vi "Accelerometer_Standalone.vi"() -> ()   [LabVIEW 2025]
uses:
  <vilib>/Instr/_visa.llb/VISA Configure Serial Port (Instr).vi
panel:
  in  "RESET":bool
  in  "Serial Port":refnum<visa-resource-name>="COM8"
  out "ACC7":cluster{"OUTX":dbl, "OUTY":dbl, "OUTZ":dbl}
  out "ACC6":cluster{"OUTX":dbl, "OUTY":dbl, "OUTZ":dbl}
  out "ACC5":cluster{"OUTX":dbl, "OUTY":dbl, "OUTZ":dbl}
  out "ACC4":cluster{"OUTX":dbl, "OUTY":dbl, "OUTZ":dbl}
  out "ACC3":cluster{"OUTX":dbl, "OUTY":dbl, "OUTZ":dbl}
  out "ACC2":cluster{"OUTX":dbl, "OUTY":dbl, "OUTZ":dbl}
  out "ACC1":cluster{"OUTX":dbl, "OUTY":dbl, "OUTZ":dbl}
  out "ACC0":cluster{"OUTX":dbl, "OUTY":dbl, "OUTZ":dbl}
  out "ACC7":cluster{"OUTX":dbl, "OUTY":dbl, "OUTZ":dbl}(graph)
  out "ACC6":cluster{"OUTX":dbl, "OUTY":dbl, "OUTZ":dbl}(graph)
  out "ACC5":cluster{"OUTX":dbl, "OUTY":dbl, "OUTZ":dbl}(graph)
  out "ACC4":cluster{"OUTX":dbl, "OUTY":dbl, "OUTZ":dbl}(graph)
  out "ACC3":cluster{"OUTX":dbl, "OUTY":dbl, "OUTZ":dbl}(graph)
  out "ACC2":cluster{"OUTX":dbl, "OUTY":dbl, "OUTZ":dbl}(graph)
  out "ACC1":cluster{"OUTX":dbl, "OUTY":dbl, "OUTZ":dbl}(graph)
  out "ACC0":cluster{"OUTX":dbl, "OUTY":dbl, "OUTZ":dbl}(graph)
  in  "Z7":dbl
  in  "Y7":dbl
  in  "X7":dbl
  in  "Z6":dbl
  in  "Y6":dbl
  in  "X6":dbl
  in  "Z5":dbl
  in  "Y5":dbl
  in  "X5":dbl
  in  "Z4":dbl=0.9
  in  "Y4":dbl=-0.18
  in  "X4":dbl=-0.05
  in  "Z3":dbl=0.9
  in  "Y3":dbl
  in  "X3":dbl
  in  "Z2":dbl=0.7
  in  "Y2":dbl=0.55
  in  "X2":dbl=0.05
  in  "Z1":dbl
  in  "Y1":dbl
  in  "X1":dbl
  in  "Z0":dbl
  in  "Y0":dbl
  in  "X0":dbl
  out "error out":errorcluster
  in  "Continous Run":bool=TRUE
  # "ACC 1 Correction Factor"
  # "ACC 0 Correction Factor"
  # "ACC 3 Correction Factor"
  # "ACC 2 Correction Factor"
  # "ACC 5 Correction Factor"
  # "ACC 4 Correction Factor"
  # "ACC 7 Correction Factor"
  # "ACC 6 Correction Factor"
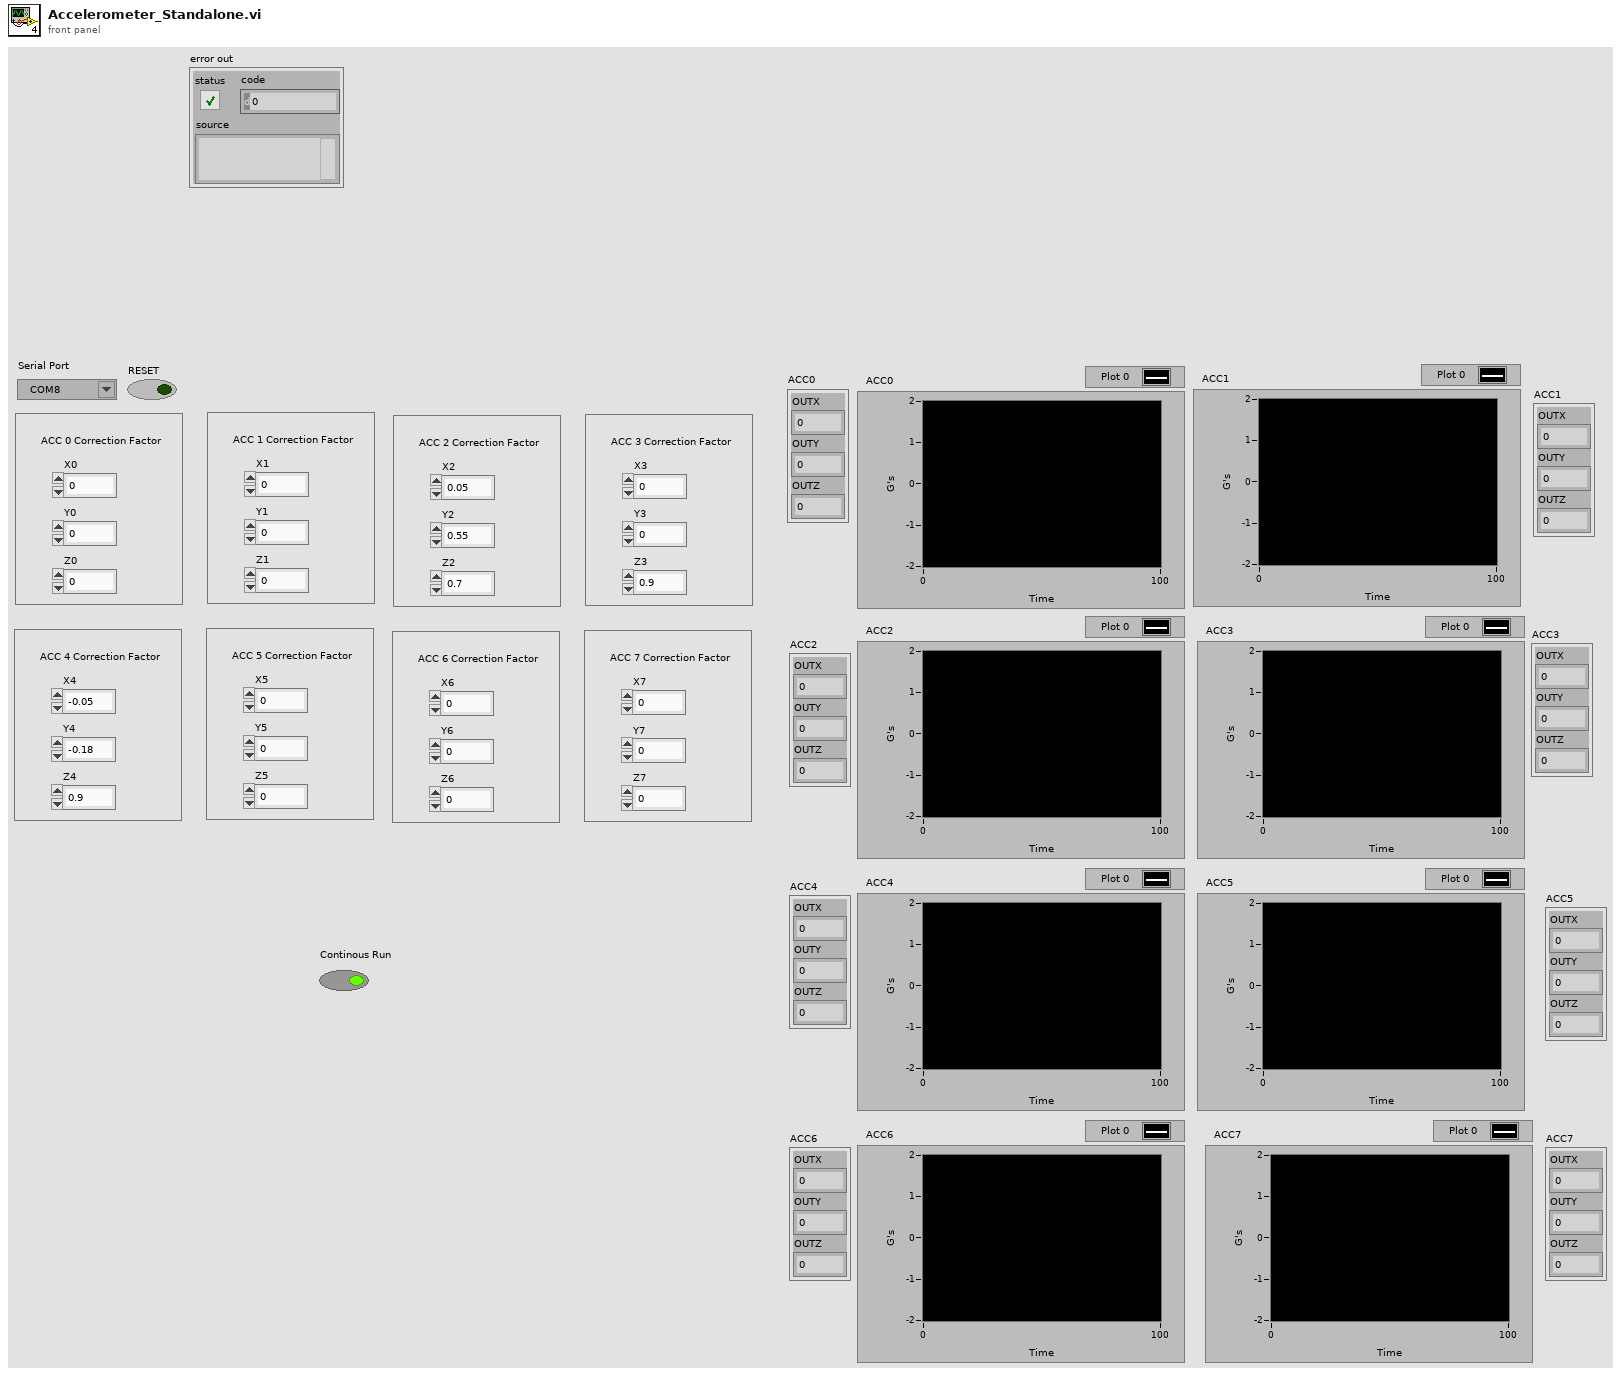
[diagram p1: front panel]
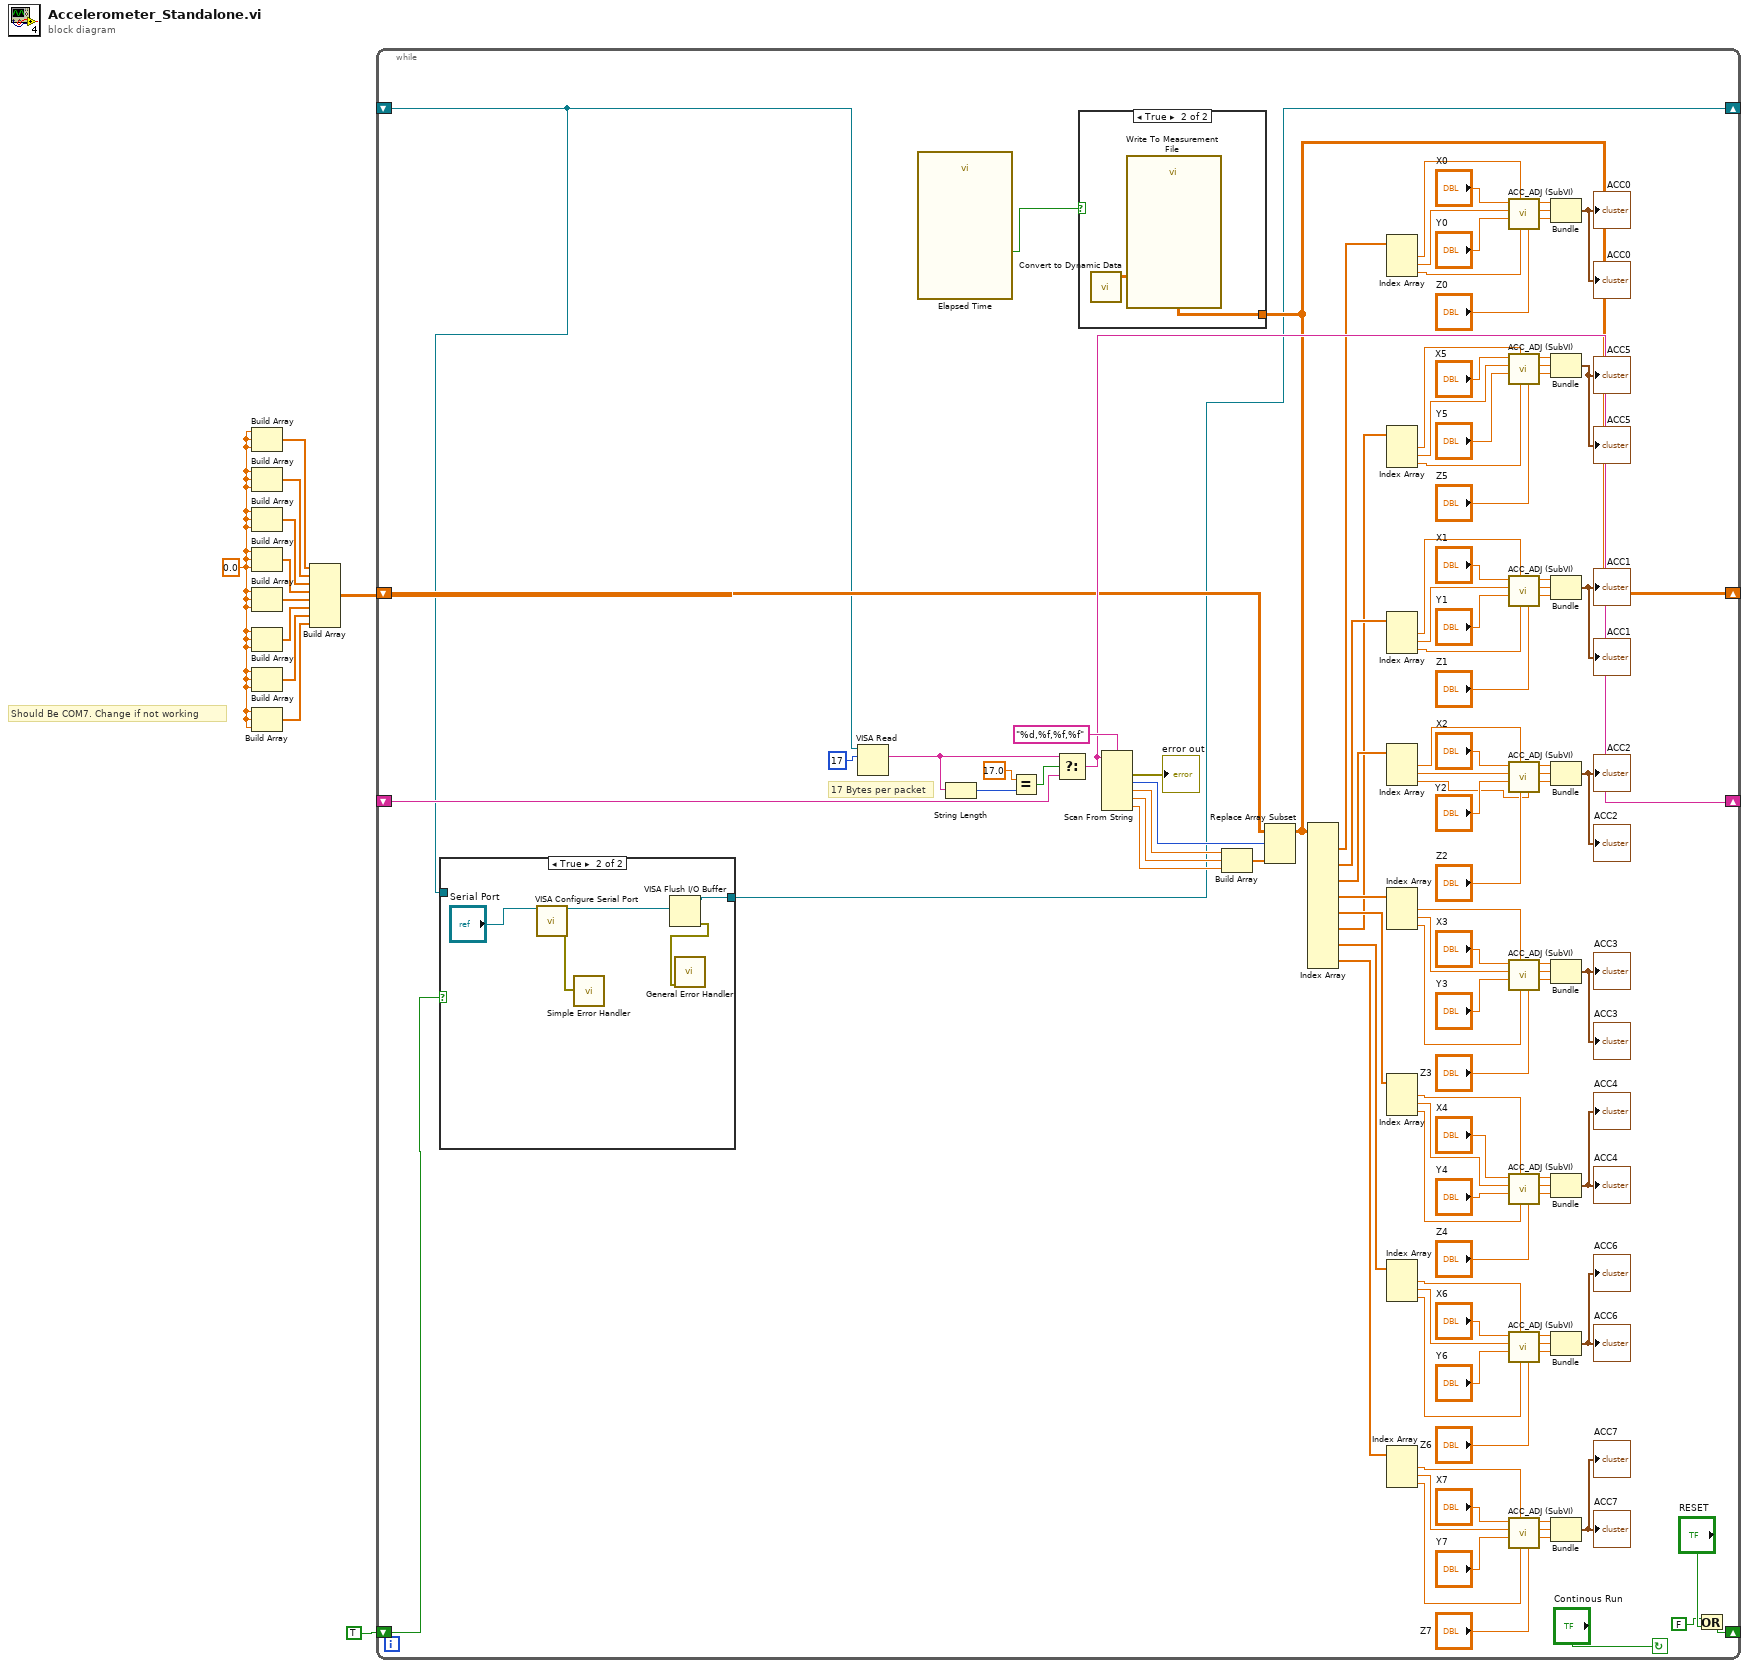
[diagram p0: block diagram]
diagram:
  w11 = 0.0 ("element")
  # "Should Be COM7. Change if not working"
  n1 = Build Array(w11, w11, w11) -> (w10:dbl[])
  n2 = Build Array(w11, w11, w11) -> (w9:dbl[])
  n3 = Build Array(w11, w11, w11) -> (w8:dbl[])
  n4 = Build Array(w11, w11, w11) -> (w7:dbl[])
  n5 = Build Array(w11, w11, w11) -> (w6:dbl[])
  n6 = Build Array(w11, w11, w11) -> (w5:dbl[])
  n7 = Build Array(w11, w11, w11) -> (w4:dbl[])
  n8 = Build Array(w11, w11, w11) -> (w3:dbl[])
  n9 = Build Array(w10, w9, w8, w7, w6, w5, w4, w3) -> (w2:dbl[][])
  n10 = while {
    shift-right: [w115] -> _
    shift-left: _ -> [w117]
    shift-right: [w19] -> _
    shift-left: w2 -> [w108]
    shift-right: [w13] -> _
    shift-left: TRUE -> [w17]
    shift-right: [w16] -> _
    shift-left: _ -> [w15]
    stop <- "Continous Run" continue-if-true
    # "17 Bytes per packet"
    n11 = case shown="True" w17 {
      tunnel: [w124 w126] -> w16
      tunnel: w15 -> [w124 _]
      frame False {
      }
      frame True {
        n12 = call-poly "VISA Configure Serial Port"("VISA resource name"="Serial Port") -> ("VISA resource name out"=w127:refnum<visa-resource-name>, "error out"=w128:errorcluster)  [unwired: 13 in]
        n13 = call <vilib>:"Simple Error Handler.vi"("error in (no error)"=w128) -> ()  [unwired: 4 in, 5 out]
        n14 = VISA Flush I/O Buffer(VISA resource name=w127) -> (VISA resource name out=w126:refnum<visa-resource-name>, error out=w125:errorcluster)  [unwired: 2 in]
        n15 = call <vilib>:"General Error Handler.vi"("error in (no error)"=w125) -> ()  [unwired: 10 in, 5 out]
      }
    }
    n16 = VISA Read(VISA resource name=w15, byte count=u32 17) -> (read buffer=w118:string)  [unwired: 1 in, 3 out]
    n17 = call "Elapsed Time"() -> ("Time has Elapsed"=w18:bool)  [unwired: 12 in, 7 out]
    n18 = String Length(string=w118) -> (length=w120:i32)
    n19 = Equal?(x=17.0, y=w120) -> (x = y?=w119:bool)
    n20 = Select(t=w118, s=w119, f=w117) -> (s? t:f=w115:string)
    n21 = Scan From String(format string="%d,%f,%f,%f", input string=w115) -> (error out=→"error out":errorcluster, output 1=w111:i32, output 2=w114:dbl, output 3=w113:dbl, output 4=w112:dbl)  [unwired: 6 in, 2 out]
    n22 = Build Array(w114, w113, w112) -> (w110:dbl[])
    n23 = Replace Array Subset(array=w108, new element=w110, index (row)=w111) -> (w19:dbl[][])  [unwired: 1 in]
    n24 = case shown="True" w18 {
      tunnel: w19 -> [_ w131]
      frame False {
      }
      frame True {
        n25 = call "Convert to Dynamic Data"("2D Array"=w131) -> ("Dynamic Data Type"=w130:dynamicdata)  [unwired: 3 in]
        n26 = call "Write To Measurement File"("Signals"=w130) -> ()  [unwired: 16 in, 3 out]
      }
    }
    n27 = Index Array(array=w19) -> (element #1=w107:dbl[], element #2=w106:dbl[], element #3=w105:dbl[], element #4=w104:dbl[], element #5=w103:dbl[], element #6=w102:dbl[], element #7=w101:dbl[], element #8=w100:dbl[])  [unwired: 16 in]
    n28 = Index Array(array=w107) -> (element #1=w99:dbl, element #2=w97:dbl, element #3=w95:dbl)  [unwired: 3 in]
    n29 = Index Array(array=w102) -> (element #1=w66:dbl, element #2=w65:dbl, element #3=w64:dbl)  [unwired: 3 in]
    n30 = Index Array(array=w106) -> (element #1=w93:dbl, element #2=w91:dbl, element #3=w89:dbl)  [unwired: 3 in]
    n31 = Index Array(array=w105) -> (element #1=w87:dbl, element #2=w85:dbl, element #3=w82:dbl)  [unwired: 3 in]
    n32 = Index Array(array=w104) -> (element #1=w81:dbl, element #2=w77:dbl, element #3=w76:dbl)  [unwired: 3 in]
    n33 = Index Array(array=w103) -> (element #1=w75:dbl, element #2=w71:dbl, element #3=w70:dbl)  [unwired: 3 in]
    n34 = Index Array(array=w101) -> (element #1=w63:dbl, element #2=w62:dbl, element #3=w61:dbl)  [unwired: 3 in]
    n35 = Index Array(array=w100) -> (element #1=w54:dbl, element #2=w53:dbl, element #3=w52:dbl)  [unwired: 3 in]
    n36 = call "ACC_ADJ (SubVI).vi"("ZADJ"="Z0", "ZIN"=w95, "XIN"=w99, "YADJ"="Y0", "YIN"=w97, "XADJ"="X0") -> ("OUTZ"=w49:dbl, "OUTY"=w50:dbl, "OUTX"=w51:dbl)  [unwired: 3 in]
    n37 = call "ACC_ADJ (SubVI).vi"("ZADJ"="Z5", "ZIN"=w64, "XIN"=w66, "YADJ"="Y5", "YIN"=w65, "XADJ"="X5") -> ("OUTZ"=w34:dbl, "OUTY"=w35:dbl, "OUTX"=w36:dbl)  [unwired: 3 in]
    n38 = call "ACC_ADJ (SubVI).vi"("ZADJ"="Z1", "ZIN"=w89, "XIN"=w93, "YADJ"="Y1", "YIN"=w91, "XADJ"="X1") -> ("OUTZ"=w46:dbl, "OUTY"=w47:dbl, "OUTX"=w48:dbl)  [unwired: 3 in]
    n39 = call "ACC_ADJ (SubVI).vi"("ZADJ"=w82, "ZIN"="Z2", "XIN"=w87, "YADJ"="Y2", "YIN"=w85, "XADJ"="X2") -> ("OUTZ"=w43:dbl, "OUTY"=w44:dbl, "OUTX"=w45:dbl)  [unwired: 3 in]
    n40 = call "ACC_ADJ (SubVI).vi"("ZADJ"="Z3", "ZIN"=w76, "XIN"=w81, "YADJ"="Y3", "YIN"=w77, "XADJ"="X3") -> ("OUTZ"=w40:dbl, "OUTY"=w41:dbl, "OUTX"=w42:dbl)  [unwired: 3 in]
    n41 = call "ACC_ADJ (SubVI).vi"("ZADJ"="Z4", "ZIN"=w70, "XIN"=w75, "YADJ"="Y4", "YIN"=w71, "XADJ"="X4") -> ("OUTZ"=w37:dbl, "OUTY"=w38:dbl, "OUTX"=w39:dbl)  [unwired: 3 in]
    n42 = call "ACC_ADJ (SubVI).vi"("ZADJ"="Z6", "ZIN"=w61, "XIN"=w63, "YADJ"="Y6", "YIN"=w62, "XADJ"="X6") -> ("OUTZ"=w31:dbl, "OUTY"=w32:dbl, "OUTX"=w33:dbl)  [unwired: 3 in]
    n43 = call "ACC_ADJ (SubVI).vi"("ZADJ"="Z7", "ZIN"=w52, "XIN"=w54, "YADJ"="Y7", "YIN"=w53, "XADJ"="X7") -> ("OUTZ"=w28:dbl, "OUTY"=w29:dbl, "OUTX"=w30:dbl)  [unwired: 3 in]
    n44 = Bundle("OUTX"=w51, "OUTY"=w50, "OUTZ"=w49) -> (→"ACC0" →"ACC0":cluster{"OUTX":dbl, "OUTY":dbl, "OUTZ":dbl})  [unwired: 1 in]
    n45 = Bundle("OUTX"=w36, "OUTY"=w35, "OUTZ"=w34) -> (→"ACC5" →"ACC5":cluster{"OUTX":dbl, "OUTY":dbl, "OUTZ":dbl})  [unwired: 1 in]
    n46 = Bundle("OUTX"=w48, "OUTY"=w47, "OUTZ"=w46) -> (→"ACC1" →"ACC1":cluster{"OUTX":dbl, "OUTY":dbl, "OUTZ":dbl})  [unwired: 1 in]
    n47 = Bundle("OUTX"=w45, "OUTY"=w44, "OUTZ"=w43) -> (→"ACC2" →"ACC2":cluster{"OUTX":dbl, "OUTY":dbl, "OUTZ":dbl})  [unwired: 1 in]
    n48 = Bundle("OUTX"=w42, "OUTY"=w41, "OUTZ"=w40) -> (→"ACC3" →"ACC3":cluster{"OUTX":dbl, "OUTY":dbl, "OUTZ":dbl})  [unwired: 1 in]
    n49 = Bundle("OUTX"=w39, "OUTY"=w38, "OUTZ"=w37) -> (→"ACC4" →"ACC4":cluster{"OUTX":dbl, "OUTY":dbl, "OUTZ":dbl})  [unwired: 1 in]
    n50 = Bundle("OUTX"=w33, "OUTY"=w32, "OUTZ"=w31) -> (→"ACC6" →"ACC6":cluster{"OUTX":dbl, "OUTY":dbl, "OUTZ":dbl})  [unwired: 1 in]
    n51 = Bundle("OUTX"=w30, "OUTY"=w29, "OUTZ"=w28) -> (→"ACC7" →"ACC7":cluster{"OUTX":dbl, "OUTY":dbl, "OUTZ":dbl})  [unwired: 1 in]
    n52 = Or(x=FALSE, y="RESET") -> (x .or. y?=w13:bool)
  }
